vi "UT - Saving Different Types.vi"(11 "index":i32) -> (0 "create error":errorcluster, 1 "write error":errorcluster, 3 "Data out":variant)   [LabVIEW 2019, in "HDF5 Tools.lvlib"]
uses:
  HDF5 Tools.lvlib
  TestClass.lvclass
  <vilib>/UPVI/lvhdf5/library.llb/HDF5 Ref.ctl
  <vilib>/UPVI/lvhdf5/dataset.llb/Simple H5Dread.xnode
  <vilib>/Utility/miscctls.llb/LVRectTypeDef.ctl
  <vilib>/UPVI/lvhdf5/file.llb/H5Fopen.vi
  <vilib>/UPVI/lvhdf5/group.llb/H5G_obj_t.ctl
  <vilib>/UPVI/lvhdf5/dataset.llb/LVH5D Operation.ctl
  <vilib>/UPVI/lvhdf5/file.llb/LVH5F Operation.ctl
  <vilib>/UPVI/lvhdf5/utility.llb/Select HDF5 Dialog.vi
  <vilib>/UPVI/lvhdf5/utility.llb/Select HDF5 Dialog (File and Object).vi
  <vilib>/UPVI/lvhdf5/utility.llb/Select HDF5 Dialog (Object Only).vi
  <vilib>/UPVI/lvhdf5/identifier.llb/Not an HDF5 Refnum Constant.vi
  <vilib>/UPVI/lvhdf5/dataset.llb/Simple H5Dread (Variant).vi
  <vilib>/UPVI/lvhdf5/dataset.llb/OpenCreateReplace Dataset.vi
  <vilib>/UPVI/lvhdf5/dataset.llb/H5Dget_space.vi
  <vilib>/UPVI/lvhdf5/dataspace.llb/H5Sget_simple_extent_dims.vi
  <vilib>/UPVI/lvhdf5/dataspace.llb/H5Sselect_hyperslab.vi
  <vilib>/UPVI/lvhdf5/dataset.llb/H5Dread (Variant).vi
  <vilib>/UPVI/lvhdf5/attribute.llb/private/LVH5AreadWDTAttrs.vi
  <vilib>/UPVI/lvhdf5/dataspace.llb/H5Sclose.vi
  <vilib>/Utility/error.llb/Error Cluster From Error Code.vi
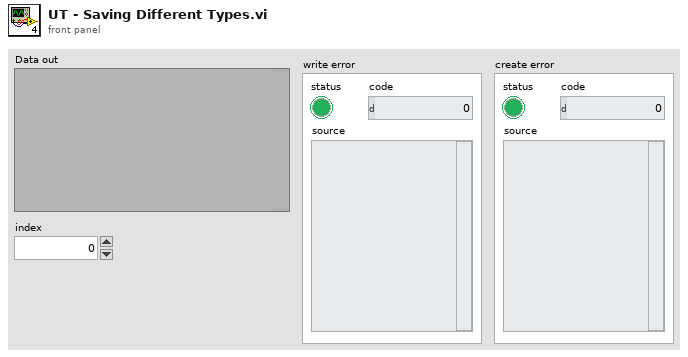
[diagram p1: front panel]
types:
  T1 = cluster{"Value":i32, "Cluster":cluster{"-Label with.dot":refnum<class "TestClass.lvclass">}}
  T2 = typedef "LVRectTypeDef.ctl" = cluster{"Left":i16, "Top":i16, "Right":i16, "Bottom":i16}
  T3 = cluster{"Behavior":enum32{"Invalid", "Default", "Floating", "Floating/Auto-Hide", "Modal"}, "Position":T2, "Center":bool, "Title":string}
  T4 = typedef "LVH5D Operation.ctl" = enum16{"open", "replace", "create", "open or create", "create or replace", "create or replace with confirmation"}
  T5 = typedef "LVH5F Operation.ctl" = enum16{"open", "open or create", "create or replace", "create or replace (with confirmation)", "create", "open (read only)"}
  T6 = typedef "H5G_obj_t.ctl" = i32
  T7 = cluster{"Object Types (any)":T6[], "Object Pattern":string}
  T8 = typedef "HDF5 Ref.ctl" = refnum<k1>
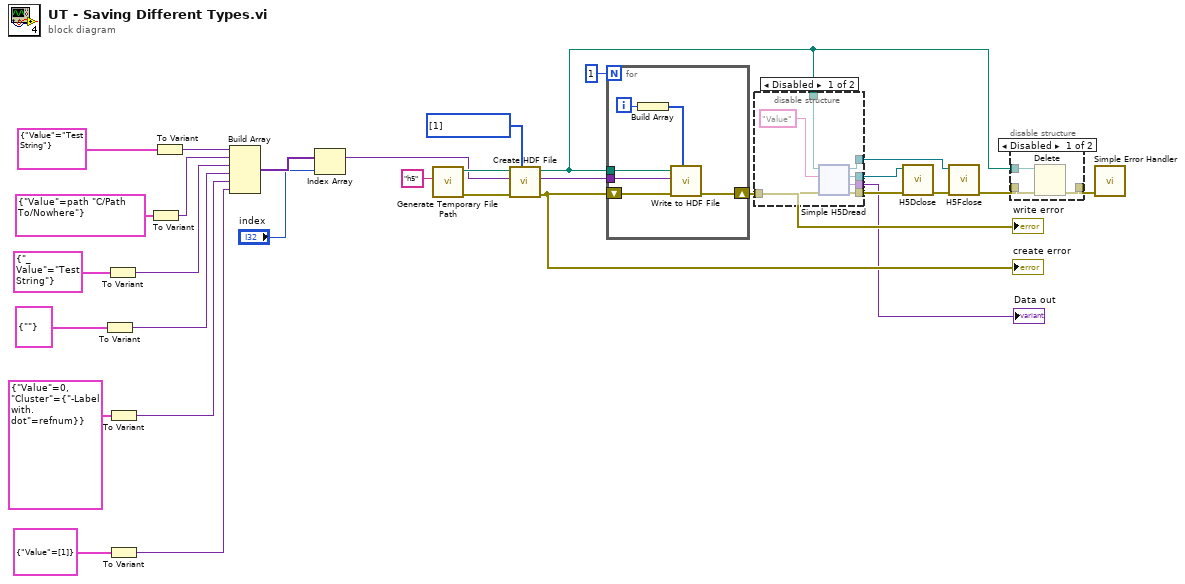
[diagram p0: block diagram]
diagram:
  n1 = To Variant(anything=cluster{"Value":string} {"Value"=""}) -> (Variant=w3:variant)
  n2 = To Variant(anything=cluster{"_Value":string} {"_Value"="Test String"}) -> (Variant=w7:variant)
  n3 = To Variant(anything=T1 {"Value"=0, "Cluster"={"-Label with.dot"=refnum}}) -> (Variant=w5:variant)
  n4 = To Variant(anything=cluster{"Value":i32[]} {"Value"=[1]}) -> (Variant=w1:variant)
  n5 = To Variant(anything=cluster{"Value":path} {"Value"=path "C:/Path To/Nowhere"}) -> (Variant=w25:variant)
  n6 = To Variant(anything=cluster{"Value":string} {"Value"="Test String"}) -> (Variant=w26:variant)
  n7 = Build Array(w26, w25, w7, w3, w5, w1) -> (w30:variant[])
  n8 = Index Array(array=w30, index="index") -> (element=w12:variant)
  n9 = call <vilib>:"Generate Temporary File Path.vi"("Temporary File Extension (tmp)"="h5") -> ("error out"=w21:errorcluster, "Unique Temporary File Path"=w22:path)  [unwired: 9 in]
  n10 = call "Create HDF File.vi"("Dims"=u64[] [1], "error in (no error)"=w21, "variant"=w12, "path"=w22) -> ("error out"=w29:errorcluster, "variant out"=w23:variant, "path out"=w10:path)  [unwired: 5 in]
  "create error" <- w29
  n11 = for {
    N: 1 -> [_]
    tunnel: w23 -> [w36]
    tunnel: w10 -> [w34]
    shift-right: [w35] -> w18
    shift-left: w29 -> [w37]
    i -> [w33]
    n12 = Build Array(w33) -> (w32:i32[])
    n13 = call "Write to HDF File.vi"("indices"=w32, "error in (no error)"=w37, "variant"=w36, "path"=w34) -> ("error out"=w35:errorcluster)  [unwired: 7 in]
  }
  "write error" <- w18
  n14 = disable-structure shown="Disabled" {
    disable-tunnel: w18 -> [w44 _]
    disable-tunnel: [w43 _] -> w17
    disable-tunnel: [w42 _] -> w14
    disable-tunnel: [w41 _] -> w13
    disable-tunnel: [w39 _] -> w11
    disable-tunnel: w10 -> [w38 _]
    frame Disabled {
      n15 = xnode "Simple H5Dread"("Dataset Path"="Value", "error in (no error)"=w44, "HDF5 Path or Ref"=w38) -> ("HDF5 Dataset Ref out"=w42:T8, "HDF5 Ref out"=w41:T8, "error out"=w43:errorcluster, "Data out"=w39:variant)  [unwired: 1 in]
    }
    frame Enabled {
    }
  }
  "Data out" <- w11
  n16 = call <vilib>:"H5Dclose.vi"("error in (no error)"=w17, "HDF5 Dataset Ref"=w14) -> ("error out"=w16:errorcluster)  [unwired: 7 in]
  n17 = call <vilib>:"H5Fclose.vi"("error in (no error)"=w16, "HDF5 Ref"=w13) -> ("error out"=w15:errorcluster)  [unwired: 7 in]
  n18 = disable-structure shown="Disabled" {
    disable-tunnel: [w363 _] -> w28
    disable-tunnel: w15 -> [w362 _]
    disable-tunnel: w10 -> [w361 _]
    frame Disabled {
      n19 = Delete(path (use dialog)=w361, error in=w362) -> (error out=w363:errorcluster)  [unwired: 3 in, 2 out]
    }
    frame Enabled {
    }
  }
  n20 = call <vilib>:"Simple Error Handler.vi"("error in (no error)"=w28) -> ()  [unwired: 4 in, 5 out]
